vi "AlazarSetRecordCount.vi"(3 "error in (no error)":errorcluster, 4 "Count":u32, 5 "Handle":u64) -> (0 "error out":errorcluster, 1 "Return Code":u32, 2 "Handle":u64)   [LabVIEW 2018]
doc: "Select the number of records to capture to on-board memory."
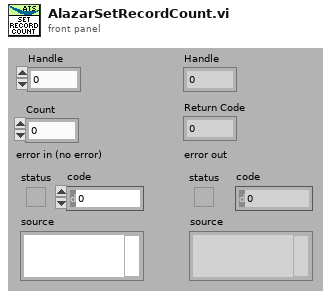
[diagram p1: front panel]
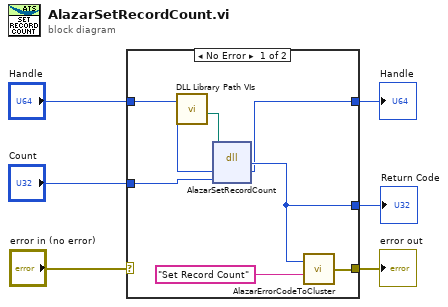
[diagram p0: block diagram]
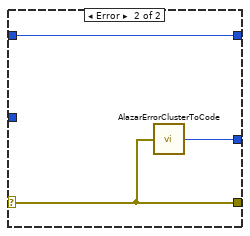
[diagram p2: hidden frame]
diagram:
  n1 = case shown="No Error" "error in (no error)" {
    selector: "error in (no error)" -> [_ w16]
    tunnel: [w10 w16] -> w5
    tunnel: [w12 w15] -> w4
    tunnel: "Handle" -> [w13 w14]
    tunnel: [w9 w14] -> w2
    tunnel: "Count" -> [w8 _]
    frame No Error {
      n2 = call "DLL Library Path VIs.vi"() -> ("Alazar"=w7:path)  [unwired: 9 in, 2 out]
      n3 = dll-call lib="C:/Project/SerialSectOCT - FFT GPU/SerialSectOCT/Labview Software/DLL/ATSApi.dll" fn="AlazarSetRecordCount"(path in=w7, "handle"=w13, "recordsPerCapture"=w8) -> ("return type"=w12:u32, "handle"=w9:u64)  [unwired: 3 in, 2 out]
      n4 = call "AlazarErrorCodeToCluster.vi"("Message"="Set Record Count", "Error Code"=w12) -> ("error out"=w10:errorcluster)
    }
    frame Error {
      n5 = call "AlazarErrorClusterToCode.vi"("error in (no error)"=w16) -> ("Error Code"=w15:u32)
    }
  }
  "Handle" <- w2
  "error out" <- w5
  "Return Code" <- w4
